vi "JsonToCluster.vi"(8 "error in (no error)":errorcluster, 11 "Telemetry in":refnum<class "Telemetry.lvclass">) -> (0 "error out":errorcluster, 3 "Telemetry out":refnum<class "Telemetry.lvclass">)   [LabVIEW 2018, in "Telemetry.lvclass"]
uses:
  Telemetry.lvclass
  Telemetry.lvclass/Telemetry.ctl
panel:
  out "error JSON":errorcluster
  # "{\n\t\"broker\": \"TCSPD160\",\n\t\"version\": \"20240131\",\n\t\"objectName\": \"               \",\n\t\"raAcquis\": \"        \",\n\t\"decAcquis\": \"        \",\n\t\"epochAcquis\": \"\",\n\t\"airMass\": \"0.000\",\n\t\"julianDate\": \"2460340.09778\",\n\t\"sideralTime\": \"        \",\n\t\"hourAngle\": \"00:00:0,\",\n\t\"date\": \"30/01/24\",\n\t\"time\": \"11:20:49\",\n\t\"rightAscention\": \"00 00 00\",\n\t\"declination\": \"00 00 00,\",\n\t\"guideStr\": \"30/01/24  00 00 00 00 00 00,\",\n\t\"guideAng\": \"   0.10\",\n\t\"guideNor\": \" 180.00\",\n\t\"guideEsp\": \"S\",\n\t\"guideCas\": \"S\",\n\t\"guidePlaca\": \"0.200\",\n\t\"statShutter\": \"\",\n\t\"posCup\": \"\",\n\t\"raOnTarget\": false,\n\t\"decOnTarget\": false,\n\t\"dome\": false,\n\t\"domeOnTarget\": false,\n\t\"guider\": false,\n\t\"mount\": false,\n\t\"grossMovement\": false,\n\t\"fineMovement\": false,\n\t\"objCentrado\": false,\n\t\"varTracking\": false,\n\t\"shutter\": false\n}"
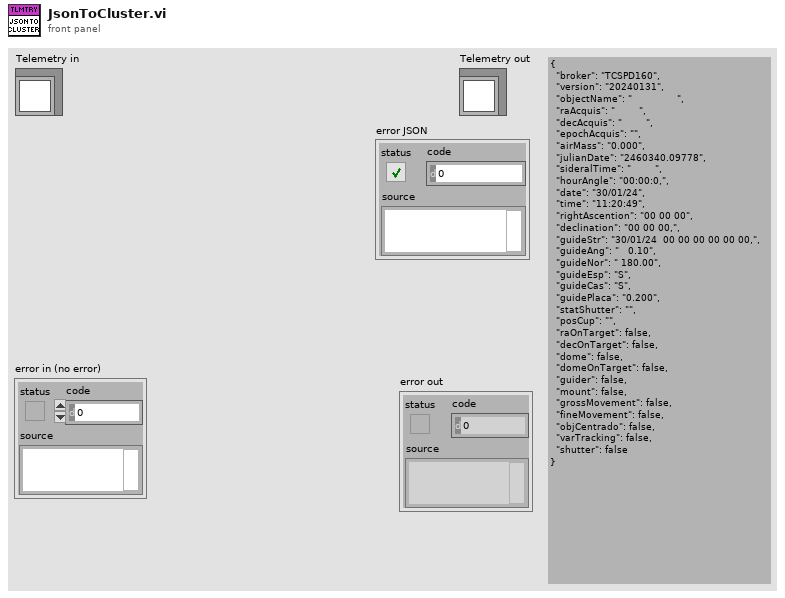
[diagram p1: front panel]
types:
  T1 = cluster{"broker":string, "version":string, "objectName":string, "raAcquis":string, "decAcquis":string, "epochAcquis":string, "airMass":string, "julianDate":string, "sideralTime":string, "hourAngle":string, "date":string, "time":string, "rightAscention":string, "declination":string, "guideStr":string, "guideAng":string, "guideNor":string, "guideEsp":string, "guideCas":string, "guidePlaca":string, "statShutter":string, "posCup":string, "raOnTarget":bool, "decOnTarget":bool, "dome":bool, "domeOnTarget":bool, "guider":bool, "mount":bool, "grossMovement":bool, "fineMovement":bool, "objCentrado":bool, "varTracking":bool, "shutter":bool, "cmd":string}
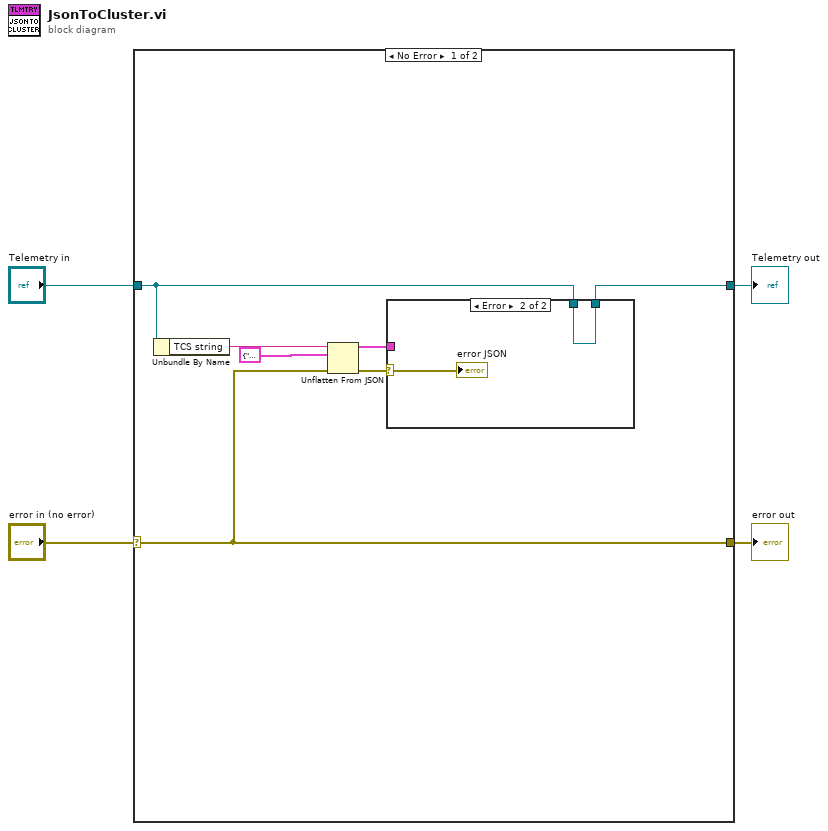
[diagram p0: block diagram]
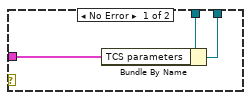
[diagram p2: hidden frame]
diagram:
  n1 = case shown="No Error" "error in (no error)" {
    selector: "error in (no error)" -> [w6 w18]
    tunnel: [w6 w18] -> w3
    tunnel: [w9 w17] -> w1
    tunnel: "Telemetry in" -> [w10 w17]
    frame No Error {
      n2 = Unbundle By Name(w10) -> ("TCS string"=w11:string)
      n3 = Unflatten From JSON(JSON string=w11, type and defaults=T1 {"broker"="", "version"="", "objectName"="", "raAcquis"="", "decAcquis"="", "epochAcquis"="", "airMass"="", "julianDate"="", "sideralTime"="", "hourAngle"="", "date"="", "time"="", "rightAscention"="", "declination"="", "guideStr"="", "guideAng"="", "guideNor"="", "guideEsp"="", "guideCas"="", "guidePlaca"="", "statShutter"="", "posCup"="", "raOnTarget"=FALSE, "decOnTarget"=FALSE, "dome"=FALSE, "domeOnTarget"=FALSE, "guider"=FALSE, "mount"=FALSE, "grossMovement"=FALSE, "fineMovement"=FALSE, "objCentrado"=FALSE, "varTracking"=FALSE, "shutter"=FALSE, "cmd"=""} ("TCS parameters"), error in (no error)=w6) -> (value=w8:T1, error out=w5:errorcluster)  [unwired: 4 in]
      n4 = case shown="Error" w5 {
        selector: w5 -> [_ w16]
        tunnel: w10 -> [w14 w15]
        tunnel: [w13 w15] -> w9
        tunnel: w8 -> [w12 _]
        frame No Error {
          n5 = Bundle By Name(cluster=w14, "TCS parameters"=w12) -> (w13:refnum<class "Telemetry.lvclass">)
        }
        frame Error {
          "error JSON" <- w16
        }
      }
    }
    frame Error {
    }
  }
  "error out" <- w3
  "Telemetry out" <- w1
